vi "get alias.vi"(8 "error in":errorcluster, 11 "configuration in":refnum<class "NISE_CEF_serializable configuration.lvclass">) -> (0 "error out":errorcluster, 2 "alias":string, 3 "configuration out":refnum<class "NISE_CEF_serializable configuration.lvclass">)   [LabVIEW 2013, in "NISE_CEF_serializable configuration.lvclass"]
uses:
  NISE_CEF_serializable configuration.lvclass
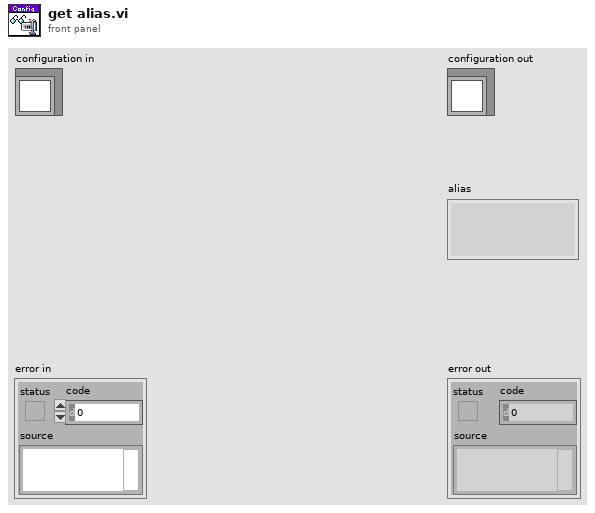
[diagram p1: front panel]
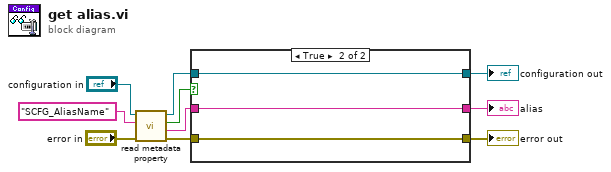
[diagram p0: block diagram]
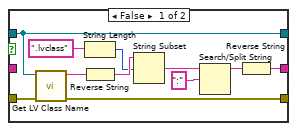
[diagram p2: hidden frame]
diagram:
  n1 = call "read metadata property.vi"("error in"="error in", "key"="SCFG_AliasName", "configuration in"="configuration in") -> ("error out"=w2:errorcluster, "value"=w6:string, "found"=w7:bool, "configuration out"=w3:refnum<class "NISE_CEF_serializable configuration.lvclass">)  [unwired: 5 in]
  n2 = case shown="True" w7 {
    tunnel: w6 -> [_ w24]
    tunnel: [w11 w24] -> w5
    tunnel: [w21 w23] -> w4
    tunnel: w3 -> [w21 w23]
    tunnel: w2 -> [w20 w22]
    tunnel: [w19 w22] -> w1
    frame False {
      n3 = call <vilib>:"Get LV Class Name.vi"("error in (no error)"=w20, "object"=w21) -> ("error out"=w19:errorcluster, "class name"=w18:string)  [unwired: 8 in]
      n4 = String Length(string=".lvclass") -> (length=w15:i32)
      n5 = Reverse String(1:w18) -> (0:w17:string)
      n6 = String Subset(string=w17, offset (0)=w15) -> (substring=w14:string)  [unwired: 1 in]
      n7 = Search/Split String(string=w14, search string/char (-)=":") -> (substring before match=w12:string)  [unwired: 1 in, 2 out]
      n8 = Reverse String(1:w12) -> (0:w11:string)
    }
    frame True {
    }
  }
  "error out" <- w1
  "configuration out" <- w4
  "alias" <- w5
